vi "ep_Read Calibration XML.vi"(8 "error in (no error)":errorcluster, 9 "nominal frequency":enum16{"50 Hz", "60 Hz"}(ring), 10 "wiring":T1=enum."3xUph + 4xI", 11 "XML file path":path) -> (0 "error out":errorcluster, 3 "calibration coefficients":T2)   [LabVIEW 2013]
uses:
  <vilib>/addons/Electrical Power/Example Support/PQ/Calibration/ep_Calibration.ctl
  <vilib>/addons/Electrical Power/PQ/Common/Controls/ep_Wiring.ctl
  <vilib>/Utility/xml.llb/Read From XML File(string).vi
  <vilib>/addons/Electrical Power/PQ/NI_EP_Power Quality.lvlib
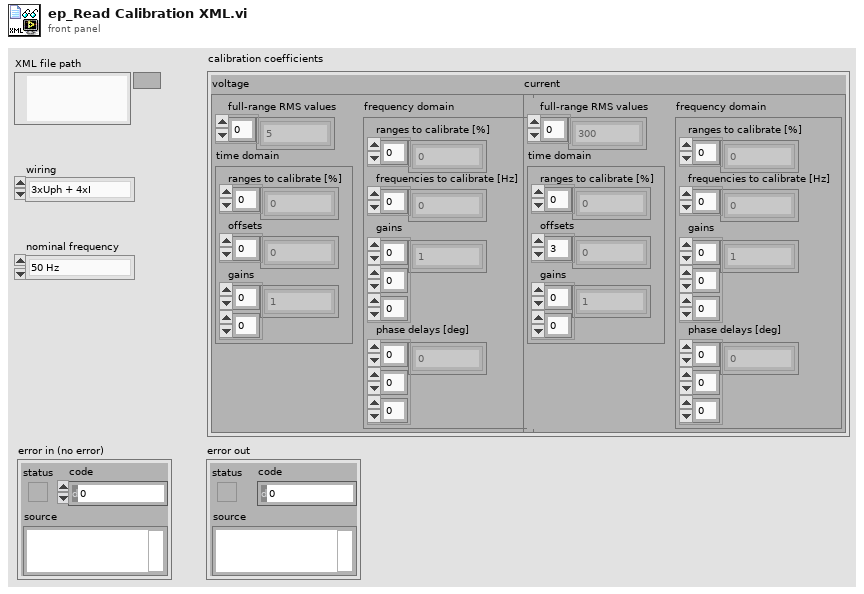
[diagram p1: front panel]
types:
  T1 = typedef "NI_EP_Power Quality.lvlib/ep_Wiring.ctl" = enum16{"4xUph + 4xI", "3xUph + 4xI", "3xUline + 4xI", "3xUph + 3xI", "3xUline + 3xI", "3xUph + 2xI", "3xUline + 2xI", "1xUph + 1xI"}
  T2 = typedef "ep_Calibration.ctl" = cluster{"voltage":cluster{"full-range RMS values":dbl[], "time domain":cluster{"ranges to calibrate [%]":dbl[], "offsets":dbl[], "gains":dbl[][]}, "frequency domain":cluster{"ranges to calibrate [%]":dbl[], "frequencies to calibrate [Hz]":dbl[], "phase delays [deg]":dbl[][][], "gains":dbl[][][]}}, "current":cluster{"full-range RMS values":dbl[], "time domain":cluster{"ranges to calibrate [%]":dbl[], "offsets":dbl[], "gains":dbl[][]}, "frequency domain":cluster{"ranges to calibrate [%]":dbl[], "frequencies to calibrate [Hz]":dbl[], "phase delays [deg]":dbl[][][], "gains":dbl[][][]}}}
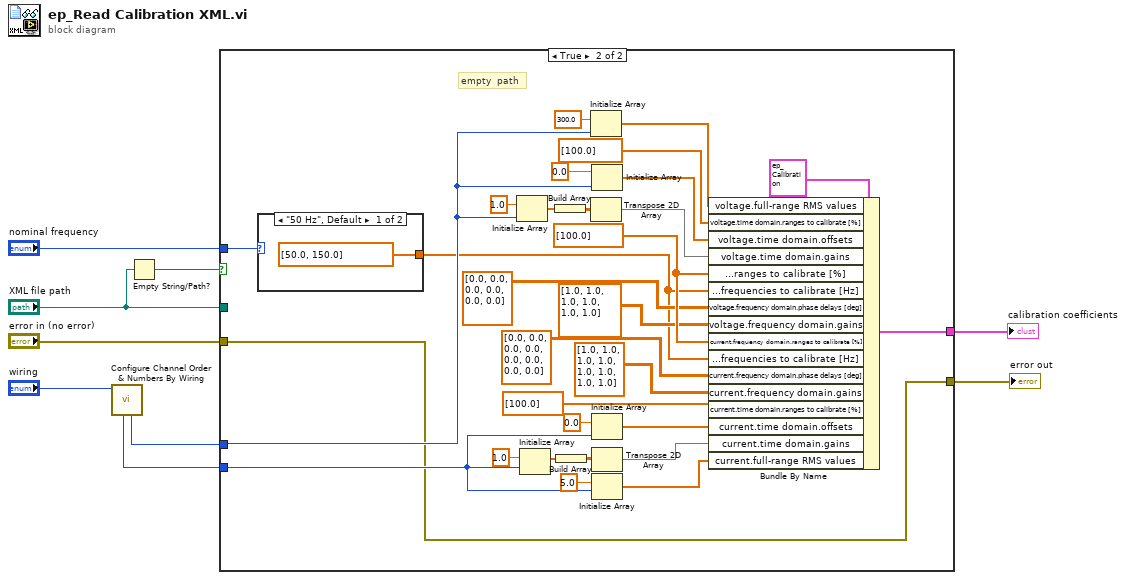
[diagram p0: block diagram]
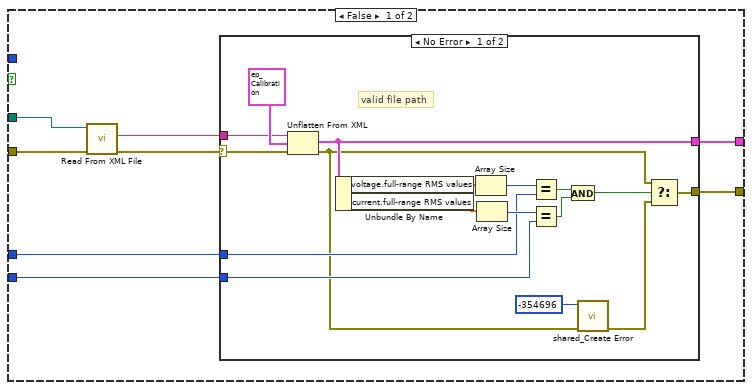
[diagram p2: hidden frame]
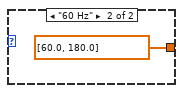
[diagram p4: hidden frame]
diagram:
  n1 = call <vilib>:"Configure Channel Order & Numbers By Wiring.vi"("wiring"="wiring") -> ("voltage#"=w3:i32, "current#"=w2:i32)  [unwired: 6 in, 3 out]
  n2 = Empty String/Path?(string/path="XML file path") -> (empty?=w7:bool)
  n3 = case shown="True" w7 {
    tunnel: [w14 w38] -> w8
    tunnel: [w17 w45] -> w9
    tunnel: w3 -> [w16 w44]
    tunnel: w2 -> [w15 w50]
    tunnel: "error in (no error)" -> [w13 w38]
    tunnel: "XML file path" -> [w12 _]
    tunnel: "nominal frequency" -> [_ w37]
    frame False {
      n4 = call-poly <vilib>:"Read From XML File.vi"("error in (no error)"=w13, "XML File Path"=w12) -> ("error out"=w10:errorcluster, "XML Elements"=w11:string)  [unwired: 7 in, 1 out]
      n5 = case shown="No Error" w10 {
        selector: w10 -> [w18 w35]
        tunnel: [w33 _] -> w17
        tunnel: w16 -> [w28 _]
        tunnel: w15 -> [w27 _]
        tunnel: [w23 w35] -> w14
        tunnel: w11 -> [w19 _]
        frame No Error {
          # "valid file path"
          n6 = Unflatten From XML(xml string=w19, type=T2 {"voltage"={"full-range RMS values"=[300.0, 300.0, 300.0], "time domain"={"ranges to calibrate [%]"=[100.0], "offsets"=[0.0, 0.0, 0.0], "gains"=[[1.0], [1.0], [1.0]]}, "frequency domain"={"ranges to calibrate [%]"=[100.0], "frequencies to calibrate [Hz]"=[50.0], "phase delays [deg]"=[[[0.0]], [[0.0]], [[0.0]]], "gains"=[[[1.0]], [[1.0]], [[1.0]]]}}, "current"={"full-range RMS values"=[5.0, 5.0, 5.0, 5.0], "time domain"={"ranges to calibrate [%]"=[100.0], "offsets"=[0.0, 0.0, 0.0, 0.0], "gains"=[[1.0], [1.0], [1.0], [1.0]]}, "frequency domain"={"ranges to calibrate [%]"=[100.0], "frequencies to calibrate [Hz]"=[50.0], "phase delays [deg]"=[[[0.0]], [[0.0]], [[0.0]], [[0.0]]], "gains"=[[[1.0]], [[1.0]], [[1.0]], [[1.0]]]}}} ("Calibration"), error in (no error)=w18) -> (value=w33:T2, error out=w20:errorcluster)
          n7 = Unbundle By Name(w33) -> ("voltage.full-range RMS values"=w32:dbl[], "current.full-range RMS values"=w31:dbl[])
          n8 = Array Size(array=w32) -> (size(s)=w29:i32)
          n9 = Array Size(array=w31) -> (size(s)=w30:i32)
          n10 = Equal?(x=w29, y=w28) -> (x = y?=w26:bool)
          n11 = Equal?(x=w30, y=w27) -> (x = y?=w25:bool)
          n12 = And(x=w26, y=w25) -> (x .and. y?=w24:bool)
          n13 = call <vilib>:"shared_Create Error.vi"("error in (no error)"=w20, "error code (0)"=-354696) -> ("error out"=w21:errorcluster)  [unwired: 9 in]
          n14 = Select(t=w20, s=w24, f=w21) -> (s? t:f=w23:errorcluster)
        }
        frame Error {
          # "invalid file path"
        }
      }
    }
    frame True {
      w57 = dbl[] [100.0] ("range percentages")
      # "empty  path"
      n15 = case shown="\"50 Hz\", Default" w37 {
        tunnel: [dbl[] [50.0, 150.0] ("frequencies to correct") dbl[] [60.0, 180.0] ("frequencies to correct")] -> w36
        frame "50 Hz", Default {
        }
        frame "60 Hz" {
        }
      }
      n16 = Initialize Array(1.0, w44) -> (w43:dbl[])
      n17 = Initialize Array(1.0 ("Numeric"), w50) -> (w48:dbl[])
      n18 = Build Array(w43) -> (w42:dbl[][])
      n19 = Build Array(w48) -> (w47:dbl[][])
      n20 = Initialize Array(300.0 ("Numeric"), w44) -> (w63:dbl[])
      n21 = Transpose 2D Array(2D array=w42) -> (transposed array=w41:dbl[][])
      n22 = Initialize Array(0.0 ("Numeric"), w44) -> (w60:dbl[])
      n23 = Initialize Array(0.0 ("Numeric"), w50) -> (w52:dbl[])
      n24 = Transpose 2D Array(2D array=w47) -> (transposed array=w46:dbl[][])
      n25 = Initialize Array(5.0 ("Numeric"), w50) -> (w54:dbl[])
      n26 = Bundle By Name(cluster=T2 {"voltage"={"full-range RMS values"=[], "time domain"={"ranges to calibrate [%]"=[], "offsets"=[], "gains"=[]}, "frequency domain"={"ranges to calibrate [%]"=[], "frequencies to calibrate [Hz]"=[], "phase delays [deg]"=[], "gains"=[]}}, "current"={"full-range RMS values"=[], "time domain"={"ranges to calibrate [%]"=[], "offsets"=[], "gains"=[]}, "frequency domain"={"ranges to calibrate [%]"=[], "frequencies to calibrate [Hz]"=[], "phase delays [deg]"=[], "gains"=[]}}} ("Calibration"), "voltage.full-range RMS values"=w63, "voltage.time domain.ranges to calibrate [%]"=dbl[] [100.0] ("range percentages"), "voltage.time domain.offsets"=w60, "voltage.time domain.gains"=w41, "voltage.frequency domain.ranges to calibrate [%]"=w57, "voltage.frequency domain.frequencies to calibrate [Hz]"=w36, "voltage.frequency domain.phase delays [deg]"=dbl[][][] [[[0.0], [0.0]], [[0.0], [0.0]], [[0.0], [0.0]]] ("phase correction"), "voltage.frequency domain.gains"=dbl[][][] [[[1.0], [1.0]], [[1.0], [1.0]], [[1.0], [1.0]]] ("amplitude correction"), "current.frequency domain.ranges to calibrate [%]"=w57, "current.frequency domain.frequencies to calibrate [Hz]"=w36, "current.frequency domain.phase delays [deg]"=dbl[][][] [[[0.0], [0.0]], [[0.0], [0.0]], [[0.0], [0.0]], [[0.0], [0.0]]] ("phase correction"), "current.frequency domain.gains"=dbl[][][] [[[1.0], [1.0]], [[1.0], [1.0]], [[1.0], [1.0]], [[1.0], [1.0]]] ("amplitude correction"), "current.time domain.ranges to calibrate [%]"=dbl[] [100.0] ("range percentages"), "current.time domain.offsets"=w52, "current.time domain.gains"=w46, "current.full-range RMS values"=w54) -> (w45:T2)
    }
  }
  "calibration coefficients" <- w9
  "error out" <- w8
